vi "Outside Connected Terminal.vi"(10 "ClassType":string, 11 "Terminal Ref In":refnum<vi>) -> (2 "Ref":refnum<vi>, 3 "Terminal Ref":refnum<vi>, 5 "Found?":bool)   [LabVIEW 2022 SP3, in "FlexBlocks Support.lvlib"]
uses:
  FlexBlocks Support.lvlib
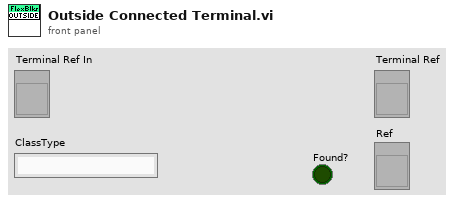
[diagram p1: front panel]
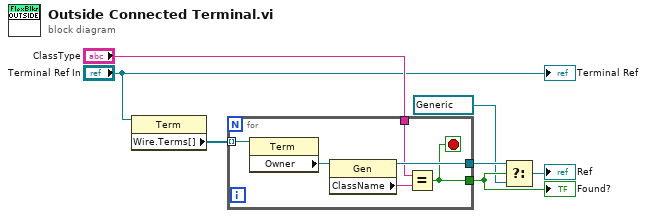
[diagram p0: block diagram]
diagram:
  n1 = property class="Term"(reference="Terminal Ref In") -> ("Wire.Terms[]"=w7:refnum<vi>[])  [unwired: 1 in, 2 out]
  n2 = for {
    tunnel: w7 -> [w11] mode=indexing
    tunnel: "ClassType" -> [w9]
    tunnel: [w10] -> w5
    tunnel: [w8] -> w4
    stop <- w8 stop-if-true
    n3 = property class="Term"(reference=w11) -> ("Owner"=w13:refnum<vi>)  [unwired: 1 in, 2 out]
    n4 = property class="Gen"(reference=w13) -> (reference out=w10:refnum<vi>, "ClassName"=w12:string)  [unwired: 1 in, 1 out]
    n5 = Equal?(x=w9, y=w12) -> (x = y?=w8:bool)
  }
  "Found?" <- w4
  n6 = Select(t=w5, s=w4, f=refnum<vi> refnum) -> (s? t:f=→"Ref":refnum<vi>)
  "Terminal Ref" <- "Terminal Ref In"
